vi "JPARC_foil_main.vi"() -> ()   [LabVIEW 2017]
uses:
  <vilib>/express/express arith-compare/Formula/XNode/ExpressFormulaBlockNode.xnode
  istr.lib/Agilent 33XXX Series/Agilent 33XXX Series.lvlib
panel:
  in  "Tab Control":enum32{"Main", "Debugging "}(tab)
  out "dt":dbl=0.05
  in  "Stop degauss":bool
  out "Counter":i32=600
  out "Waveform Chart":dbl(graph)
  in  "order":i64=2
  in  "Start Degauss":bool
  in  "T_end (s)":dbl=30.0 format="%_5f"
  in  "T_period (s)":dbl=1.0 format="%_5f"
  in  "I_max_d (A)":dbl=10.0 format="%_5f"
  in  "Set curet (A)":dbl min=0.0 max=120.0 format="%_5f"
  in  "OUTPUT":bool
  in  "stop":bool
  in  "I_lim_up (A)":dbl=10.1 format="%_5f"
  in  "I_lim_low (A)":dbl=-0.1 format="%_5f"
  out "Graph (Set current)":cluster{timestamp[], dbl[]}(graph)={[timestamp(3707259196.4848704 s since 1904-01-01), timestamp(3707259199.20108 s since 1904-01-01), timestamp(3707259200.17246 s since 1904-01-01), timestamp(3707259200.2159233 s since 1904-01-01), timestamp(3707259200.28732 s since 1904-01-01), timestamp(3707259200.328816 s since 1904-01-01), timestamp(3707259200.377073 s since 1904-01-01), timestamp(3707259200.420492 s since 1904-01-01), timestamp(3707259200.467496 s since 1904-01-01), timestamp(3707259200.518796 s since 1904-01-01), timestamp(3707259200.570331 s since 1904-01-01), timestamp(3707259200.620787 s since 1904-01-01), timestamp(3707259200.672 s since 1904-01-01), timestamp(3707259200.7227407 s since 1904-01-01), timestamp(3707259200.7737064 s since 1904-01-01), timestamp(3707259200.8259854 s since 1904-01-01), timestamp(3707259200.8772697 s since 1904-01-01), timestamp(3707259200.9277143 s since 1904-01-01), timestamp(3707259200.979037 s since 1904-01-01), timestamp(3707259201.0299745 s since 1904-01-01), timestamp(3707259201.081536 s since 1904-01-01), timestamp(3707259201.13187 s since 1904-01-01), timestamp(3707259201.182979 s since 1904-01-01), timestamp(3707259201.2563944 s since 1904-01-01), timestamp(3707259201.299408 s since 1904-01-01), timestamp(3707259201.342004 s since 1904-01-01), timestamp(3707259201.3879175 s since 1904-01-01), timestamp(3707259201.4399514 s since 1904-01-01), timestamp(3707259201.4893274 s since 1904-01-01), timestamp(3707259201.5397305 s since 1904-01-01), timestamp(3707259201.5915103 s since 1904-01-01), timestamp(3707259201.6417384 s since 1904-01-01), timestamp(3707259201.693012 s since 1904-01-01), timestamp(3707259201.7436895 s since 1904-01-01), timestamp(3707259201.7946744 s since 1904-01-01), timestamp(3707259201.845514 s since 1904-01-01), timestamp(3707259201.8961496 s since 1904-01-01), timestamp(3707259201.9476814 s since 1904-01-01), timestamp(3707259201.999445 s since 1904-01-01), timestamp(3707259202.0498457 s since 1904-01-01), timestamp(3707259202.101092 s since 1904-01-01), timestamp(3707259202.152056 s since 1904-01-01), timestamp(3707259202.204391 s since 1904-01-01), timestamp(3707259202.2552943 s since 1904-01-01), timestamp(3707259202.305813 s since 1904-01-01), timestamp(3707259202.3572016 s since 1904-01-01), timestamp(3707259202.408192 s since 1904-01-01), timestamp(3707259202.458596 s since 1904-01-01), timestamp(3707259202.5099535 s since 1904-01-01), timestamp(3707259202.56095 s since 1904-01-01), timestamp(3707259202.6127977 s since 1904-01-01), timestamp(3707259202.6857367 s since 1904-01-01), timestamp(3707259202.727055 s since 1904-01-01), timestamp(3707259202.77362 s since 1904-01-01), timestamp(3707259202.818931 s since 1904-01-01), timestamp(3707259202.8698378 s since 1904-01-01), timestamp(3707259202.921864 s since 1904-01-01), timestamp(3707259202.9730167 s since 1904-01-01), timestamp(3707259203.0247264 s since 1904-01-01), timestamp(3707259203.0752497 s since 1904-01-01), timestamp(3707259203.1262217 s since 1904-01-01), timestamp(3707259203.1771607 s since 1904-01-01), timestamp(3707259203.2284536 s since 1904-01-01), timestamp(3707259203.279292 s since 1904-01-01), timestamp(3707259203.3309326 s since 1904-01-01), timestamp(3707259203.3821626 s since 1904-01-01), timestamp(3707259203.4327054 s since 1904-01-01), timestamp(3707259203.4840465 s since 1904-01-01), timestamp(3707259203.5348983 s since 1904-01-01), timestamp(3707259203.586394 s since 1904-01-01), timestamp(3707259203.636896 s since 1904-01-01), timestamp(3707259203.687648 s since 1904-01-01), timestamp(3707259203.7388554 s since 1904-01-01), timestamp(3707259203.7898073 s since 1904-01-01), timestamp(3707259203.8409944 s since 1904-01-01), timestamp(3707259203.8924065 s since 1904-01-01), timestamp(3707259203.9434342 s since 1904-01-01), timestamp(3707259203.994741 s since 1904-01-01), timestamp(3707259204.046955 s since 1904-01-01), timestamp(3707259204.0980425 s since 1904-01-01), timestamp(3707259204.1488814 s since 1904-01-01), timestamp(3707259204.200164 s since 1904-01-01), timestamp(3707259204.2748857 s since 1904-01-01), timestamp(3707259204.321075 s since 1904-01-01), timestamp(3707259204.364665 s since 1904-01-01), timestamp(3707259204.410939 s since 1904-01-01), timestamp(3707259204.462568 s since 1904-01-01), timestamp(3707259204.513267 s since 1904-01-01), timestamp(3707259204.5636735 s since 1904-01-01), timestamp(3707259204.6150465 s since 1904-01-01), timestamp(3707259204.666663 s since 1904-01-01), timestamp(3707259204.7179313 s since 1904-01-01), timestamp(3707259204.7687726 s since 1904-01-01), timestamp(3707259204.819624 s since 1904-01-01), timestamp(3707259204.870779 s since 1904-01-01), timestamp(3707259204.922157 s since 1904-01-01), timestamp(3707259204.9727407 s since 1904-01-01), timestamp(3707259205.0238824 s since 1904-01-01), timestamp(3707259205.0761695 s since 1904-01-01), timestamp(3707259205.127436 s since 1904-01-01), timestamp(3707259205.177644 s since 1904-01-01), timestamp(3707259205.230016 s since 1904-01-01), timestamp(3707259205.281155 s since 1904-01-01), timestamp(3707259205.3321023 s since 1904-01-01), timestamp(3707259205.384508 s since 1904-01-01), timestamp(3707259205.4351106 s since 1904-01-01), timestamp(3707259205.4859486 s since 1904-01-01), timestamp(3707259205.537502 s since 1904-01-01), timestamp(3707259205.587603 s since 1904-01-01), timestamp(3707259205.6386504 s since 1904-01-01), timestamp(3707259205.69032 s since 1904-01-01), timestamp(3707259205.74035 s since 1904-01-01), timestamp(3707259205.791466 s since 1904-01-01), timestamp(3707259205.8418894 s since 1904-01-01), timestamp(3707259205.8925257 s since 1904-01-01), timestamp(3707259205.9429784 s since 1904-01-01), timestamp(3707259205.993564 s since 1904-01-01), timestamp(3707259206.043586 s since 1904-01-01), timestamp(3707259206.0935864 s since 1904-01-01), timestamp(3707259206.14396 s since 1904-01-01), timestamp(3707259206.194829 s since 1904-01-01), timestamp(3707259206.2456946 s since 1904-01-01), timestamp(3707259206.3135138 s since 1904-01-01), timestamp(3707259206.3546143 s since 1904-01-01), timestamp(3707259206.4024615 s since 1904-01-01), timestamp(3707259206.4513326 s since 1904-01-01), timestamp(3707259206.5024624 s since 1904-01-01), timestamp(3707259206.5528274 s since 1904-01-01), timestamp(3707259206.6034446 s since 1904-01-01), timestamp(3707259206.653367 s since 1904-01-01), timestamp(3707259206.705113 s since 1904-01-01), timestamp(3707259206.754691 s since 1904-01-01), timestamp(3707259206.806076 s since 1904-01-01), timestamp(3707259206.857049 s since 1904-01-01), timestamp(3707259206.9079337 s since 1904-01-01), timestamp(3707259206.9591393 s since 1904-01-01), timestamp(3707259207.010139 s since 1904-01-01), timestamp(3707259207.061363 s since 1904-01-01), timestamp(3707259207.1352954 s since 1904-01-01), timestamp(3707259207.1819334 s since 1904-01-01), timestamp(3707259207.227907 s since 1904-01-01), timestamp(3707259207.2730746 s since 1904-01-01), timestamp(3707259207.3175426 s since 1904-01-01), timestamp(3707259207.3691216 s since 1904-01-01), timestamp(3707259207.419863 s since 1904-01-01), timestamp(3707259207.4709153 s since 1904-01-01), timestamp(3707259207.522387 s since 1904-01-01), timestamp(3707259207.5742 s since 1904-01-01), timestamp(3707259207.626405 s since 1904-01-01), timestamp(3707259207.676672 s since 1904-01-01), timestamp(3707259207.7275534 s since 1904-01-01), timestamp(3707259207.7778554 s since 1904-01-01), timestamp(3707259207.8297663 s since 1904-01-01), timestamp(3707259207.88111 s since 1904-01-01), timestamp(3707259207.93376 s since 1904-01-01), timestamp(3707259207.9848967 s since 1904-01-01), timestamp(3707259208.0358834 s since 1904-01-01), timestamp(3707259208.087055 s since 1904-01-01), timestamp(3707259208.1377134 s since 1904-01-01), timestamp(3707259208.1888857 s since 1904-01-01), timestamp(3707259208.241416 s since 1904-01-01), timestamp(3707259208.2919464 s since 1904-01-01), timestamp(3707259208.3427296 s since 1904-01-01), timestamp(3707259208.393376 s since 1904-01-01), timestamp(3707259208.443455 s since 1904-01-01), timestamp(3707259208.4941254 s since 1904-01-01), timestamp(3707259208.5451374 s since 1904-01-01), timestamp(3707259208.596422 s since 1904-01-01), timestamp(3707259208.647224 s since 1904-01-01), timestamp(3707259208.6983647 s since 1904-01-01), timestamp(3707259208.748924 s since 1904-01-01), timestamp(3707259208.800724 s since 1904-01-01), timestamp(3707259208.851848 s since 1904-01-01), timestamp(3707259208.904263 s since 1904-01-01), timestamp(3707259208.954531 s since 1904-01-01), timestamp(3707259209.0045705 s since 1904-01-01), timestamp(3707259209.056037 s since 1904-01-01), timestamp(3707259209.107112 s since 1904-01-01), timestamp(3707259209.1579194 s since 1904-01-01), timestamp(3707259209.2093368 s since 1904-01-01), timestamp(3707259209.260172 s since 1904-01-01), timestamp(3707259209.311596 s since 1904-01-01), timestamp(3707259209.362818 s since 1904-01-01), timestamp(3707259209.4141088 s since 1904-01-01), timestamp(3707259209.4664073 s since 1904-01-01), timestamp(3707259209.517049 s since 1904-01-01), timestamp(3707259209.56796 s since 1904-01-01), timestamp(3707259209.6186466 s since 1904-01-01), timestamp(3707259209.6698775 s since 1904-01-01), timestamp(3707259209.721443 s since 1904-01-01), timestamp(3707259209.771893 s since 1904-01-01), timestamp(3707259209.8232145 s since 1904-01-01), timestamp(3707259209.87515 s since 1904-01-01), timestamp(3707259209.9262233 s since 1904-01-01), timestamp(3707259209.9767776 s since 1904-01-01), timestamp(3707259210.0292993 s since 1904-01-01), timestamp(3707259210.0800896 s since 1904-01-01), timestamp(3707259210.1313114 s since 1904-01-01), timestamp(3707259210.1819234 s since 1904-01-01), timestamp(3707259210.2327647 s since 1904-01-01), timestamp(3707259210.283632 s since 1904-01-01), timestamp(3707259210.3363066 s since 1904-01-01), timestamp(3707259210.38682 s since 1904-01-01), timestamp(3707259210.439037 s since 1904-01-01), timestamp(3707259210.489682 s since 1904-01-01), timestamp(3707259210.5407295 s since 1904-01-01), timestamp(3707259210.592229 s since 1904-01-01), timestamp(3707259210.6426926 s since 1904-01-01), timestamp(3707259210.6941586 s since 1904-01-01), timestamp(3707259210.7443247 s since 1904-01-01), timestamp(3707259210.7950273 s since 1904-01-01), timestamp(3707259210.8457465 s since 1904-01-01), timestamp(3707259210.897409 s since 1904-01-01), timestamp(3707259210.9487 s since 1904-01-01), timestamp(3707259210.9995775 s since 1904-01-01), timestamp(3707259211.050323 s since 1904-01-01), timestamp(3707259211.101493 s since 1904-01-01), timestamp(3707259211.151855 s since 1904-01-01), timestamp(3707259211.203181 s since 1904-01-01), timestamp(3707259211.2537966 s since 1904-01-01), timestamp(3707259211.3054895 s since 1904-01-01), timestamp(3707259211.355844 s since 1904-01-01), timestamp(3707259211.4072433 s since 1904-01-01), timestamp(3707259211.4580126 s since 1904-01-01), timestamp(3707259211.5096097 s since 1904-01-01), timestamp(3707259211.560656 s since 1904-01-01), timestamp(3707259211.611928 s since 1904-01-01), timestamp(3707259211.6628976 s since 1904-01-01), timestamp(3707259211.714095 s since 1904-01-01), timestamp(3707259211.766273 s since 1904-01-01), timestamp(3707259211.8179936 s since 1904-01-01), timestamp(3707259211.869491 s since 1904-01-01), timestamp(3707259211.921025 s since 1904-01-01), timestamp(3707259211.972306 s since 1904-01-01), timestamp(3707259212.023468 s since 1904-01-01), timestamp(3707259212.0753655 s since 1904-01-01), timestamp(3707259212.126084 s since 1904-01-01), timestamp(3707259212.1770864 s since 1904-01-01), timestamp(3707259212.229044 s since 1904-01-01), timestamp(3707259212.2800536 s since 1904-01-01), timestamp(3707259212.3323584 s since 1904-01-01), timestamp(3707259212.383467 s since 1904-01-01), timestamp(3707259212.4347086 s since 1904-01-01), timestamp(3707259212.486989 s since 1904-01-01), timestamp(3707259212.53818 s since 1904-01-01), timestamp(3707259212.58933 s since 1904-01-01), timestamp(3707259212.640089 s since 1904-01-01), timestamp(3707259212.701696 s since 1904-01-01), timestamp(3707259212.7540417 s since 1904-01-01), timestamp(3707259212.8061337 s since 1904-01-01), timestamp(3707259212.8567905 s since 1904-01-01), timestamp(3707259212.9081287 s since 1904-01-01), timestamp(3707259212.9602423 s since 1904-01-01), timestamp(3707259213.0107985 s since 1904-01-01), timestamp(3707259213.063319 s since 1904-01-01), timestamp(3707259213.1145 s since 1904-01-01), timestamp(3707259213.165478 s since 1904-01-01), timestamp(3707259213.216491 s since 1904-01-01), timestamp(3707259213.267567 s since 1904-01-01), timestamp(3707259213.318584 s since 1904-01-01), timestamp(3707259213.3694696 s since 1904-01-01), timestamp(3707259213.4201455 s since 1904-01-01), timestamp(3707259213.4707623 s since 1904-01-01), timestamp(3707259213.5227647 s since 1904-01-01), timestamp(3707259213.5735393 s since 1904-01-01), timestamp(3707259213.6239495 s since 1904-01-01), timestamp(3707259213.675685 s since 1904-01-01), timestamp(3707259213.7274256 s since 1904-01-01), timestamp(3707259213.7781906 s since 1904-01-01), timestamp(3707259213.8294616 s since 1904-01-01), timestamp(3707259213.880292 s since 1904-01-01), timestamp(3707259213.9308977 s since 1904-01-01), timestamp(3707259213.982133 s since 1904-01-01), timestamp(3707259214.0334015 s since 1904-01-01), timestamp(3707259214.084085 s since 1904-01-01), timestamp(3707259214.135271 s since 1904-01-01), timestamp(3707259214.185329 s since 1904-01-01), timestamp(3707259214.2361574 s since 1904-01-01), timestamp(3707259214.287383 s since 1904-01-01), timestamp(3707259214.337472 s since 1904-01-01), timestamp(3707259214.3874817 s since 1904-01-01), timestamp(3707259214.438272 s since 1904-01-01), timestamp(3707259214.489022 s since 1904-01-01), timestamp(3707259214.540349 s since 1904-01-01), timestamp(3707259214.590536 s since 1904-01-01), timestamp(3707259214.64076 s since 1904-01-01), timestamp(3707259214.700007 s since 1904-01-01), timestamp(3707259214.7501864 s since 1904-01-01), timestamp(3707259214.8015146 s since 1904-01-01), timestamp(3707259214.8524246 s since 1904-01-01), timestamp(3707259214.9026446 s since 1904-01-01), timestamp(3707259214.954119 s since 1904-01-01), timestamp(3707259215.0048494 s since 1904-01-01), timestamp(3707259215.057986 s since 1904-01-01), timestamp(3707259215.10916 s since 1904-01-01), timestamp(3707259215.1601553 s since 1904-01-01), timestamp(3707259215.213757 s since 1904-01-01), timestamp(3707259215.265211 s since 1904-01-01), timestamp(3707259215.316068 s since 1904-01-01), timestamp(3707259215.3673697 s since 1904-01-01), timestamp(3707259215.417912 s since 1904-01-01), timestamp(3707259215.469684 s since 1904-01-01), timestamp(3707259215.520413 s since 1904-01-01), timestamp(3707259215.570737 s since 1904-01-01), timestamp(3707259215.621899 s since 1904-01-01), timestamp(3707259215.672473 s since 1904-01-01), timestamp(3707259215.7224584 s since 1904-01-01), timestamp(3707259215.773552 s since 1904-01-01), timestamp(3707259215.824029 s since 1904-01-01), timestamp(3707259215.8763375 s since 1904-01-01), timestamp(3707259215.927059 s since 1904-01-01), timestamp(3707259215.9783382 s since 1904-01-01), timestamp(3707259216.0288734 s since 1904-01-01), timestamp(3707259216.0800967 s since 1904-01-01), timestamp(3707259216.1305 s since 1904-01-01), timestamp(3707259216.1806087 s since 1904-01-01), timestamp(3707259216.2318783 s since 1904-01-01), timestamp(3707259216.283163 s since 1904-01-01), timestamp(3707259216.3337545 s since 1904-01-01), timestamp(3707259216.3863034 s since 1904-01-01), timestamp(3707259216.436903 s since 1904-01-01), timestamp(3707259216.4876494 s since 1904-01-01), timestamp(3707259216.5379634 s since 1904-01-01), timestamp(3707259216.5895176 s since 1904-01-01), timestamp(3707259216.640459 s since 1904-01-01), timestamp(3707259216.690654 s since 1904-01-01), timestamp(3707259216.742255 s since 1904-01-01), timestamp(3707259216.7949896 s since 1904-01-01), timestamp(3707259216.8460145 s since 1904-01-01), timestamp(3707259216.8970914 s since 1904-01-01), timestamp(3707259216.9476047 s since 1904-01-01), timestamp(3707259217.0005393 s since 1904-01-01), timestamp(3707259217.051352 s since 1904-01-01), timestamp(3707259217.102024 s since 1904-01-01), timestamp(3707259217.1528993 s since 1904-01-01), timestamp(3707259217.203648 s since 1904-01-01), timestamp(3707259217.256073 s since 1904-01-01), timestamp(3707259217.3070145 s since 1904-01-01), timestamp(3707259217.356732 s since 1904-01-01), timestamp(3707259217.4104424 s since 1904-01-01), timestamp(3707259217.4607873 s since 1904-01-01), timestamp(3707259217.5116177 s since 1904-01-01), timestamp(3707259217.5639296 s since 1904-01-01), timestamp(3707259217.6161304 s since 1904-01-01), timestamp(3707259217.6665506 s since 1904-01-01), timestamp(3707259217.7166615 s since 1904-01-01), timestamp(3707259217.767932 s since 1904-01-01), timestamp(3707259217.819317 s since 1904-01-01), timestamp(3707259217.8699727 s since 1904-01-01), timestamp(3707259217.9206257 s since 1904-01-01), timestamp(3707259217.9714575 s since 1904-01-01), timestamp(3707259218.021664 s since 1904-01-01), timestamp(3707259218.0726857 s since 1904-01-01), timestamp(3707259218.124248 s since 1904-01-01), timestamp(3707259218.1760406 s since 1904-01-01), timestamp(3707259218.2275505 s since 1904-01-01), timestamp(3707259218.2780695 s since 1904-01-01), timestamp(3707259218.3291097 s since 1904-01-01), timestamp(3707259218.3796663 s since 1904-01-01), timestamp(3707259218.4309096 s since 1904-01-01), timestamp(3707259218.482177 s since 1904-01-01), timestamp(3707259218.5334377 s since 1904-01-01), timestamp(3707259218.5839825 s since 1904-01-01), timestamp(3707259218.6347857 s since 1904-01-01), timestamp(3707259218.687488 s since 1904-01-01), timestamp(3707259218.7368326 s since 1904-01-01), timestamp(3707259218.7891154 s since 1904-01-01), timestamp(3707259218.840208 s since 1904-01-01), timestamp(3707259218.891742 s since 1904-01-01), timestamp(3707259218.94312 s since 1904-01-01), timestamp(3707259218.9935336 s since 1904-01-01), timestamp(3707259219.0437903 s since 1904-01-01), timestamp(3707259219.095799 s since 1904-01-01), timestamp(3707259219.155056 s since 1904-01-01), timestamp(3707259219.2061977 s since 1904-01-01), timestamp(3707259219.266284 s since 1904-01-01), timestamp(3707259219.317372 s since 1904-01-01), timestamp(3707259219.367924 s since 1904-01-01), timestamp(3707259219.4185576 s since 1904-01-01), timestamp(3707259219.4702945 s since 1904-01-01), timestamp(3707259219.520776 s since 1904-01-01), timestamp(3707259219.5729456 s since 1904-01-01), timestamp(3707259219.6249 s since 1904-01-01), timestamp(3707259219.676088 s since 1904-01-01), timestamp(3707259219.726608 s since 1904-01-01), timestamp(3707259219.7775393 s since 1904-01-01), timestamp(3707259219.8276463 s since 1904-01-01), timestamp(3707259219.8794065 s since 1904-01-01), timestamp(3707259219.9297304 s since 1904-01-01), timestamp(3707259219.981024 s since 1904-01-01), timestamp(3707259220.032031 s since 1904-01-01), timestamp(3707259220.08276 s since 1904-01-01), timestamp(3707259220.13502 s since 1904-01-01), timestamp(3707259220.186343 s since 1904-01-01), timestamp(3707259220.2370896 s since 1904-01-01), timestamp(3707259220.2879705 s since 1904-01-01), timestamp(3707259220.340339 s since 1904-01-01), timestamp(3707259220.391716 s since 1904-01-01), timestamp(3707259220.450717 s since 1904-01-01), timestamp(3707259220.503291 s since 1904-01-01), timestamp(3707259220.5555534 s since 1904-01-01), timestamp(3707259220.606714 s since 1904-01-01), timestamp(3707259220.658076 s since 1904-01-01), timestamp(3707259220.709576 s since 1904-01-01), timestamp(3707259220.759384 s since 1904-01-01), timestamp(3707259220.810531 s since 1904-01-01), timestamp(3707259220.860863 s since 1904-01-01), timestamp(3707259220.9124303 s since 1904-01-01), timestamp(3707259220.9629617 s since 1904-01-01), timestamp(3707259221.01416 s since 1904-01-01), timestamp(3707259221.0653095 s since 1904-01-01), timestamp(3707259221.115598 s since 1904-01-01), timestamp(3707259221.1672006 s since 1904-01-01), timestamp(3707259221.217863 s since 1904-01-01), timestamp(3707259221.2699904 s since 1904-01-01), timestamp(3707259221.322552 s since 1904-01-01), timestamp(3707259221.3738728 s since 1904-01-01), timestamp(3707259221.425934 s since 1904-01-01), timestamp(3707259221.477443 s since 1904-01-01), timestamp(3707259221.52782 s since 1904-01-01), timestamp(3707259221.5785017 s since 1904-01-01), timestamp(3707259221.628906 s since 1904-01-01), timestamp(3707259221.6805334 s since 1904-01-01), timestamp(3707259221.7307234 s since 1904-01-01), timestamp(3707259221.7821255 s since 1904-01-01), timestamp(3707259221.833152 s since 1904-01-01), timestamp(3707259221.883951 s since 1904-01-01), timestamp(3707259221.9346166 s since 1904-01-01), timestamp(3707259221.987086 s since 1904-01-01), timestamp(3707259222.0374384 s since 1904-01-01), timestamp(3707259222.087833 s since 1904-01-01), timestamp(3707259222.1391544 s since 1904-01-01), timestamp(3707259222.1914062 s since 1904-01-01), timestamp(3707259222.2418942 s since 1904-01-01), timestamp(3707259222.2929454 s since 1904-01-01), timestamp(3707259222.3446894 s since 1904-01-01), timestamp(3707259222.3967385 s since 1904-01-01), timestamp(3707259222.447489 s since 1904-01-01), timestamp(3707259222.497763 s since 1904-01-01), timestamp(3707259222.54918 s since 1904-01-01), timestamp(3707259222.6010094 s since 1904-01-01), timestamp(3707259222.6523314 s since 1904-01-01), timestamp(3707259222.7027655 s since 1904-01-01), timestamp(3707259222.754297 s since 1904-01-01), timestamp(3707259222.8053575 s since 1904-01-01), timestamp(3707259222.856412 s since 1904-01-01), timestamp(3707259222.9070864 s since 1904-01-01), timestamp(3707259222.958297 s since 1904-01-01), timestamp(3707259223.009618 s since 1904-01-01), timestamp(3707259223.0613146 s since 1904-01-01), timestamp(3707259223.11218 s since 1904-01-01), timestamp(3707259223.1625433 s since 1904-01-01), timestamp(3707259223.2127657 s since 1904-01-01), timestamp(3707259223.2645383 s since 1904-01-01), timestamp(3707259223.3150783 s since 1904-01-01), timestamp(3707259223.3659673 s since 1904-01-01), timestamp(3707259223.418496 s since 1904-01-01), timestamp(3707259223.4693246 s since 1904-01-01), timestamp(3707259223.5205846 s since 1904-01-01), timestamp(3707259223.570944 s since 1904-01-01), timestamp(3707259223.6216254 s since 1904-01-01), timestamp(3707259223.682088 s since 1904-01-01), timestamp(3707259223.733576 s since 1904-01-01), timestamp(3707259223.784137 s since 1904-01-01), timestamp(3707259223.83652 s since 1904-01-01), timestamp(3707259223.8887234 s since 1904-01-01), timestamp(3707259223.939524 s since 1904-01-01), timestamp(3707259223.990504 s since 1904-01-01), timestamp(3707259224.0408306 s since 1904-01-01), timestamp(3707259224.093295 s since 1904-01-01), timestamp(3707259224.1437054 s since 1904-01-01), timestamp(3707259224.19502 s since 1904-01-01), timestamp(3707259224.245454 s since 1904-01-01), timestamp(3707259224.29636 s since 1904-01-01), timestamp(3707259224.347352 s since 1904-01-01), timestamp(3707259224.398108 s since 1904-01-01), timestamp(3707259224.449426 s since 1904-01-01), timestamp(3707259224.500648 s since 1904-01-01), timestamp(3707259224.5518937 s since 1904-01-01), timestamp(3707259224.6029873 s since 1904-01-01), timestamp(3707259224.654089 s since 1904-01-01), timestamp(3707259224.706424 s since 1904-01-01), timestamp(3707259224.75725 s since 1904-01-01), timestamp(3707259224.8075743 s since 1904-01-01), timestamp(3707259224.857317 s since 1904-01-01), timestamp(3707259224.908 s since 1904-01-01), timestamp(3707259224.9592695 s since 1904-01-01), timestamp(3707259225.0099897 s since 1904-01-01), timestamp(3707259225.060612 s since 1904-01-01), timestamp(3707259225.1121006 s since 1904-01-01), timestamp(3707259225.163561 s since 1904-01-01), timestamp(3707259225.2141614 s since 1904-01-01), timestamp(3707259225.2663345 s since 1904-01-01), timestamp(3707259225.316788 s since 1904-01-01), timestamp(3707259225.3684354 s since 1904-01-01), timestamp(3707259225.419561 s since 1904-01-01), timestamp(3707259225.4698944 s since 1904-01-01), timestamp(3707259225.52236 s since 1904-01-01), timestamp(3707259225.5731654 s since 1904-01-01), timestamp(3707259225.624091 s since 1904-01-01), timestamp(3707259225.675978 s since 1904-01-01), timestamp(3707259225.727556 s since 1904-01-01), timestamp(3707259225.778472 s since 1904-01-01), timestamp(3707259225.8297086 s since 1904-01-01), timestamp(3707259225.8806744 s since 1904-01-01), timestamp(3707259225.9340096 s since 1904-01-01), timestamp(3707259225.9844646 s since 1904-01-01), timestamp(3707259226.0369096 s since 1904-01-01), timestamp(3707259226.088491 s since 1904-01-01), timestamp(3707259226.138916 s since 1904-01-01), timestamp(3707259226.1902647 s since 1904-01-01), timestamp(3707259226.241206 s since 1904-01-01), timestamp(3707259226.29248 s since 1904-01-01), timestamp(3707259226.3426905 s since 1904-01-01), timestamp(3707259226.393713 s since 1904-01-01), timestamp(3707259226.4446816 s since 1904-01-01), timestamp(3707259226.4961057 s since 1904-01-01), timestamp(3707259226.5475063 s since 1904-01-01), timestamp(3707259226.5974383 s since 1904-01-01), timestamp(3707259226.647401 s since 1904-01-01), timestamp(3707259226.6976 s since 1904-01-01), timestamp(3707259226.748803 s since 1904-01-01), timestamp(3707259226.8003407 s since 1904-01-01), timestamp(3707259226.8516073 s since 1904-01-01), timestamp(3707259226.9029126 s since 1904-01-01), timestamp(3707259226.95415 s since 1904-01-01), timestamp(3707259227.0043664 s since 1904-01-01), timestamp(3707259227.055092 s since 1904-01-01), timestamp(3707259227.1056786 s since 1904-01-01), timestamp(3707259227.15715 s since 1904-01-01), timestamp(3707259227.2084703 s since 1904-01-01), timestamp(3707259227.2600713 s since 1904-01-01), timestamp(3707259227.3114734 s since 1904-01-01), timestamp(3707259227.36184 s since 1904-01-01), timestamp(3707259227.41304 s since 1904-01-01), timestamp(3707259227.4637184 s since 1904-01-01), timestamp(3707259227.516283 s since 1904-01-01), timestamp(3707259227.5666585 s since 1904-01-01), timestamp(3707259227.617522 s since 1904-01-01), timestamp(3707259227.667171 s since 1904-01-01), timestamp(3707259227.717443 s since 1904-01-01), timestamp(3707259227.7677736 s since 1904-01-01), timestamp(3707259227.8190265 s since 1904-01-01), timestamp(3707259227.86989 s since 1904-01-01), timestamp(3707259227.9213367 s since 1904-01-01), timestamp(3707259227.972058 s since 1904-01-01), timestamp(3707259228.022944 s since 1904-01-01), timestamp(3707259228.0737743 s since 1904-01-01), timestamp(3707259228.126157 s since 1904-01-01), timestamp(3707259228.179792 s since 1904-01-01), timestamp(3707259228.230928 s since 1904-01-01), timestamp(3707259228.2822247 s since 1904-01-01), timestamp(3707259228.3334584 s since 1904-01-01), timestamp(3707259228.3851233 s since 1904-01-01), timestamp(3707259228.4358015 s since 1904-01-01), timestamp(3707259228.487086 s since 1904-01-01), timestamp(3707259228.5382576 s since 1904-01-01), timestamp(3707259228.589992 s since 1904-01-01), timestamp(3707259228.6409473 s since 1904-01-01), timestamp(3707259228.6921864 s since 1904-01-01), timestamp(3707259228.7431855 s since 1904-01-01), timestamp(3707259228.793529 s since 1904-01-01), timestamp(3707259228.8443007 s since 1904-01-01), timestamp(3707259228.895092 s since 1904-01-01), timestamp(3707259228.9469104 s since 1904-01-01), timestamp(3707259228.9980783 s since 1904-01-01), timestamp(3707259229.0492735 s since 1904-01-01), timestamp(3707259229.0995064 s since 1904-01-01), timestamp(3707259229.150301 s since 1904-01-01), timestamp(3707259229.201368 s since 1904-01-01), timestamp(3707259229.254064 s since 1904-01-01), timestamp(3707259229.3044486 s since 1904-01-01), timestamp(3707259229.3551073 s since 1904-01-01), timestamp(3707259229.4070864 s since 1904-01-01), timestamp(3707259229.457599 s since 1904-01-01), timestamp(3707259229.5088544 s since 1904-01-01), timestamp(3707259229.5599866 s since 1904-01-01), timestamp(3707259229.6109066 s since 1904-01-01), timestamp(3707259229.662153 s since 1904-01-01), timestamp(3707259229.712928 s since 1904-01-01), timestamp(3707259229.764052 s since 1904-01-01), timestamp(3707259229.815863 s since 1904-01-01), timestamp(3707259229.867405 s since 1904-01-01), timestamp(3707259229.916816 s since 1904-01-01), timestamp(3707259229.967896 s since 1904-01-01), timestamp(3707259230.020653 s since 1904-01-01), timestamp(3707259230.0722766 s since 1904-01-01), timestamp(3707259230.1225095 s since 1904-01-01), timestamp(3707259230.1731434 s since 1904-01-01), timestamp(3707259230.224079 s since 1904-01-01), timestamp(3707259230.2750993 s since 1904-01-01), timestamp(3707259230.3256216 s since 1904-01-01), timestamp(3707259230.3771567 s since 1904-01-01), timestamp(3707259230.427674 s since 1904-01-01), timestamp(3707259230.4784455 s since 1904-01-01), timestamp(3707259230.529454 s since 1904-01-01), timestamp(3707259230.5793514 s since 1904-01-01), timestamp(3707259230.629626 s since 1904-01-01), timestamp(3707259230.680669 s since 1904-01-01), timestamp(3707259230.7320294 s since 1904-01-01), timestamp(3707259230.7828393 s since 1904-01-01), timestamp(3707259230.834331 s since 1904-01-01), timestamp(3707259230.886357 s since 1904-01-01), timestamp(3707259230.936435 s since 1904-01-01)], array[604 elements]} caption="XY Graph"
  in  "VISA (Agilent 34402)":refnum<visa-resource-name>="GPIB0::15::INSTR"
  out "Agilent\nIntialized?":bool=TRUE
  in  "Initialize (Agilent)":bool
  in  "base path":path=path "C:/LabVIEW/DATA/J-PARC_202107/test_0623"
  out "time elapsed (ms)":u32=30726
  out "File Error Out":errorcluster
  out "error out (Agilent)":errorcluster
  # "GP016-10 control"
  # "Degaussing routine"
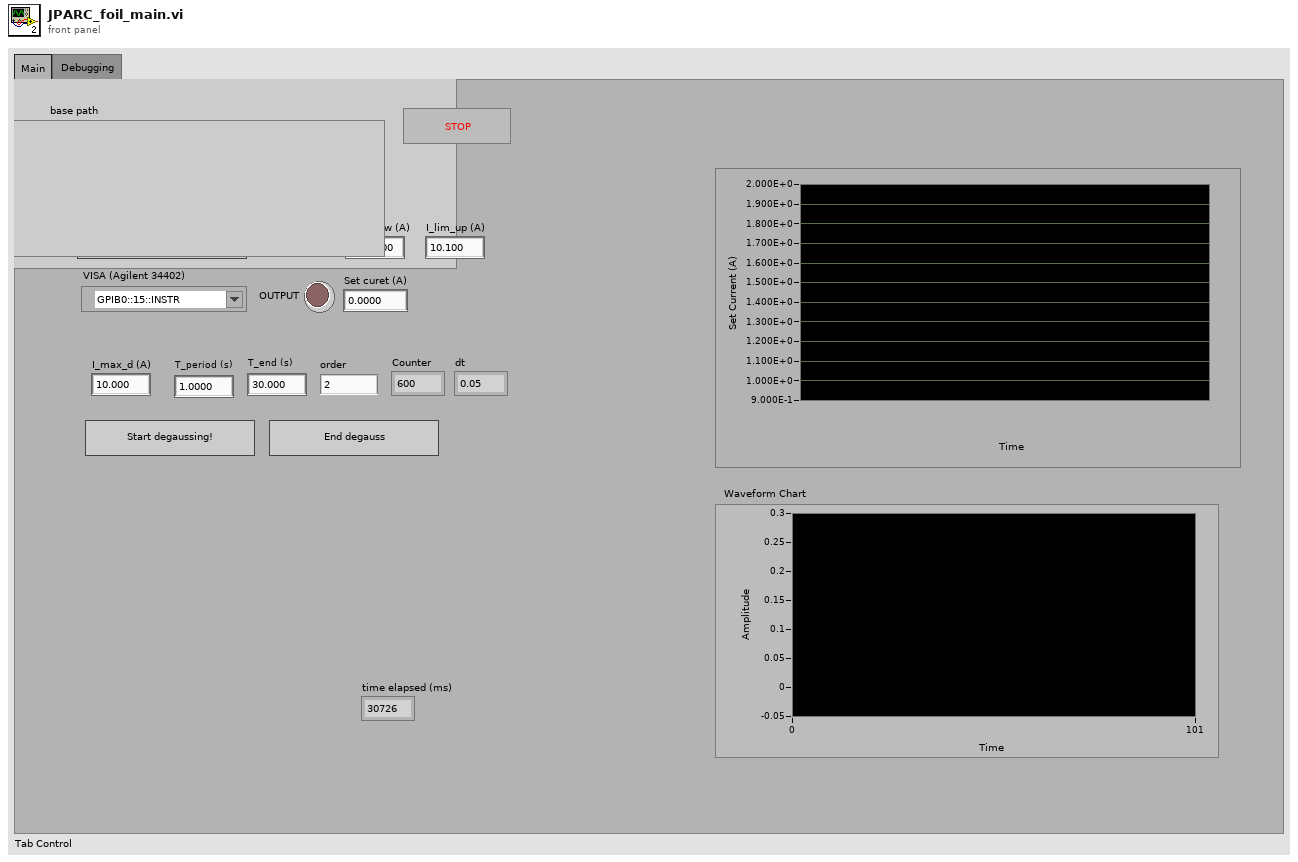
[diagram p1: front panel]
types:
  T1 = enum16{"open", "replace", "create", "open or create", "replace or create", "replace or create with confirmation"}
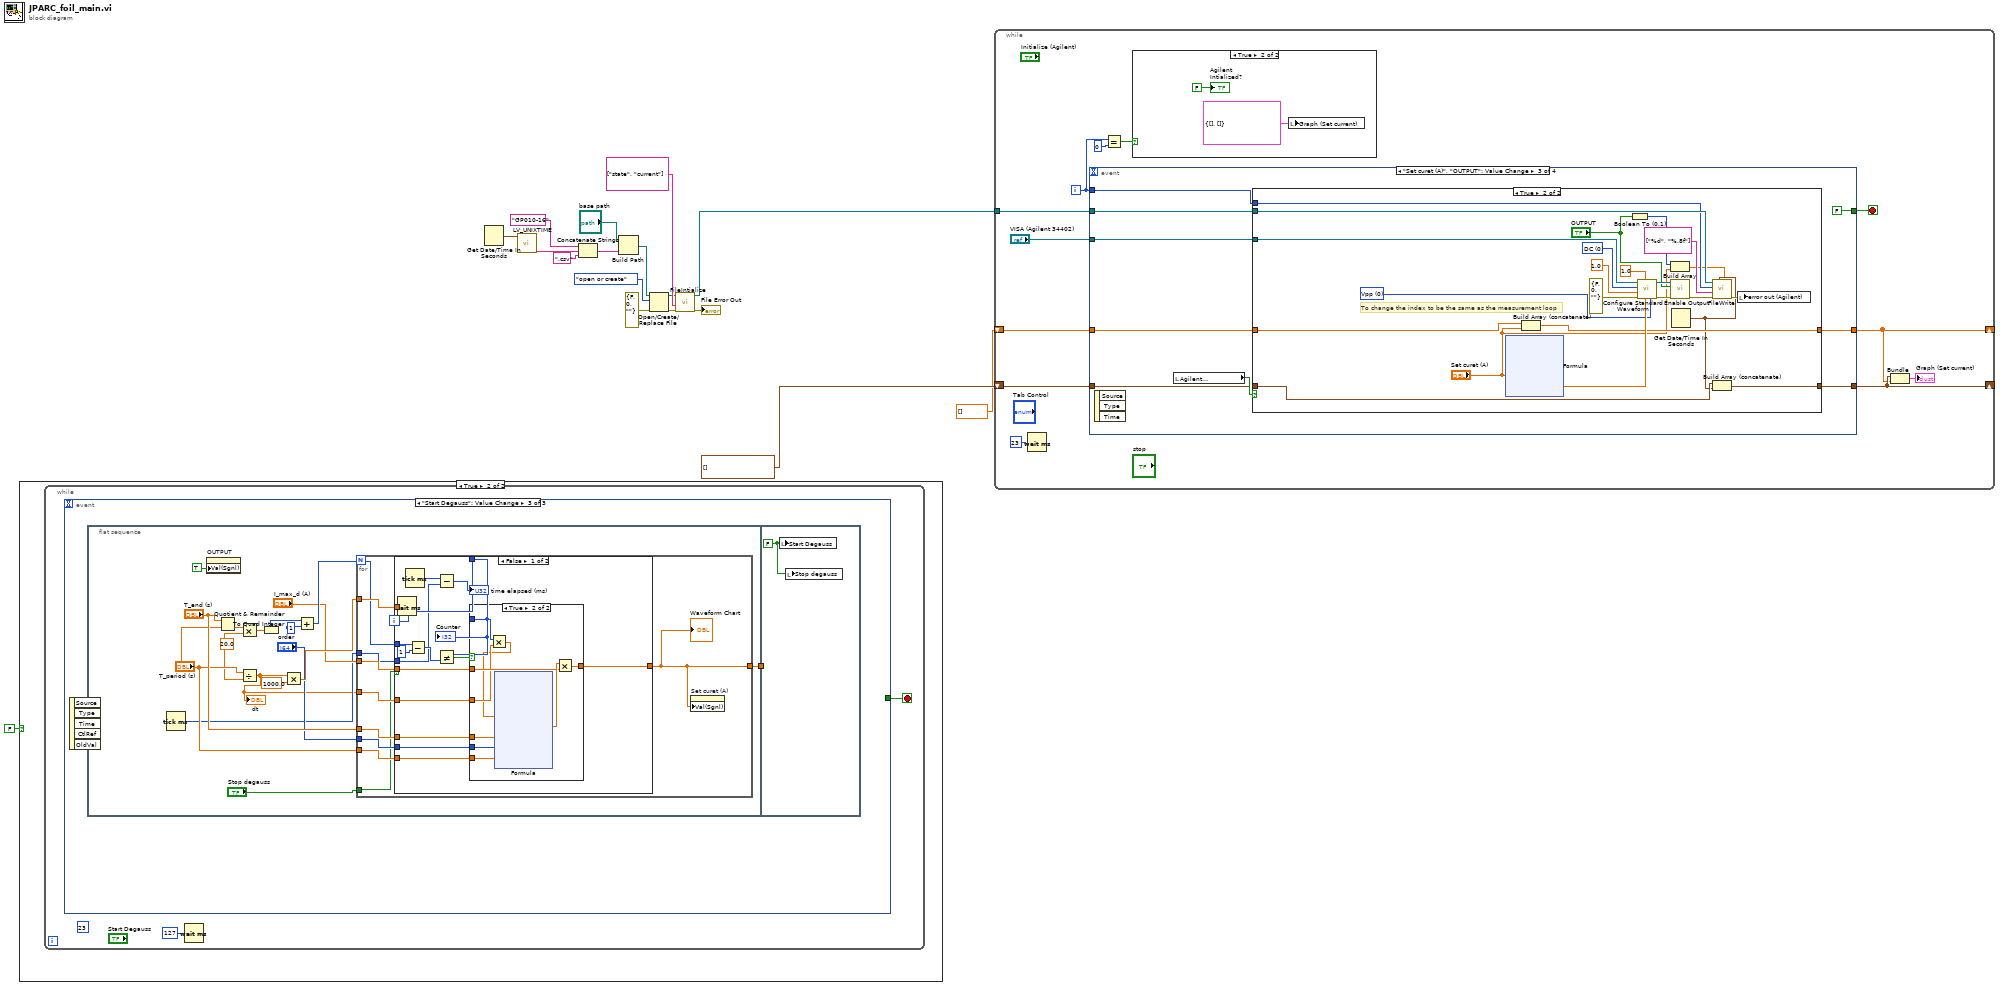
[diagram p0: block diagram]
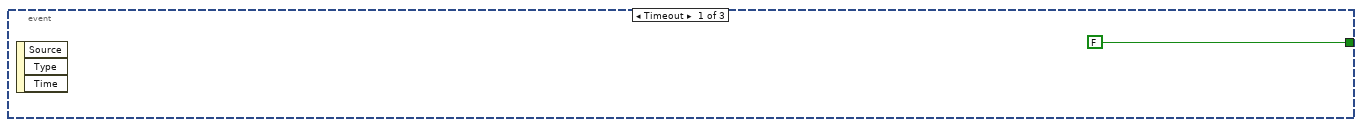
[diagram p3: hidden frame]
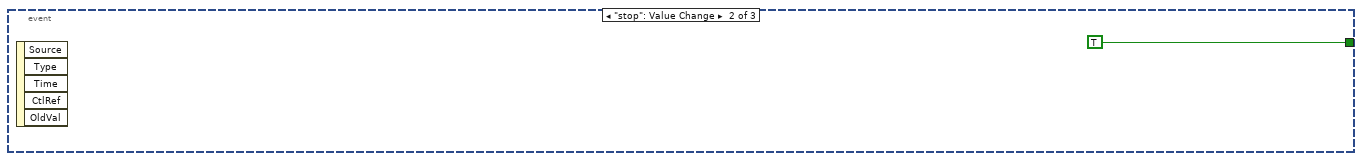
[diagram p4: hidden frame]
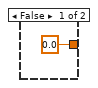
[diagram p5: hidden frame]
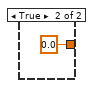
[diagram p6: hidden frame]
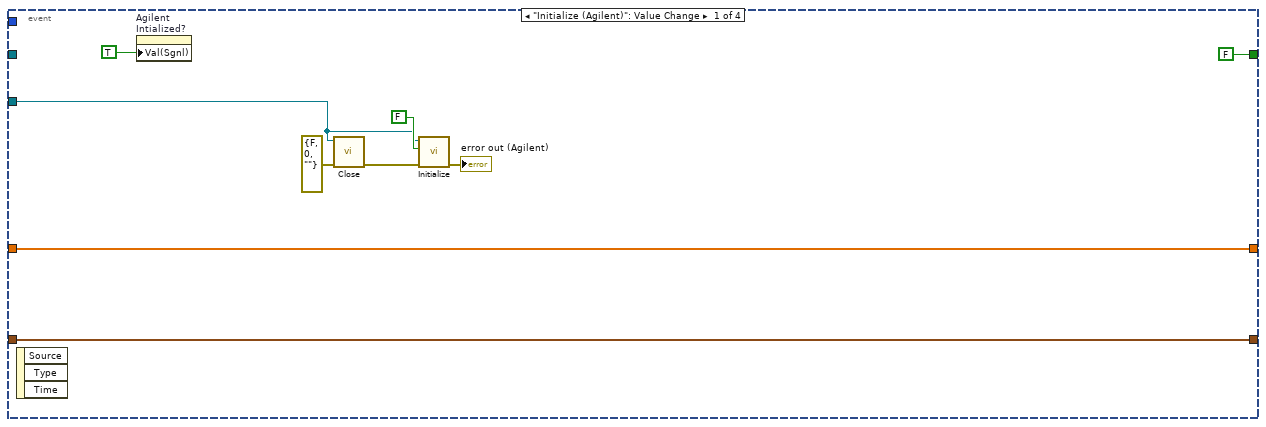
[diagram p8: hidden frame]
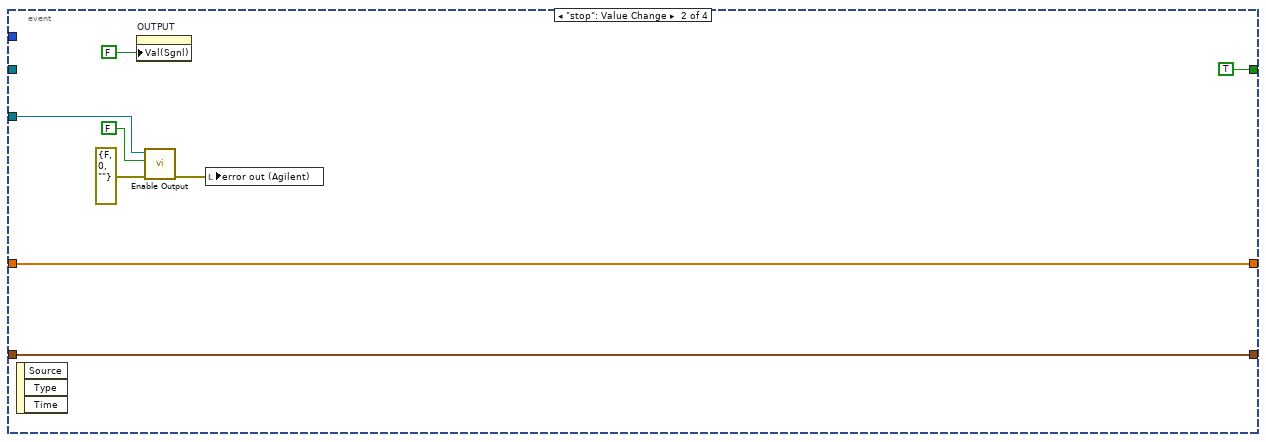
[diagram p9: hidden frame]
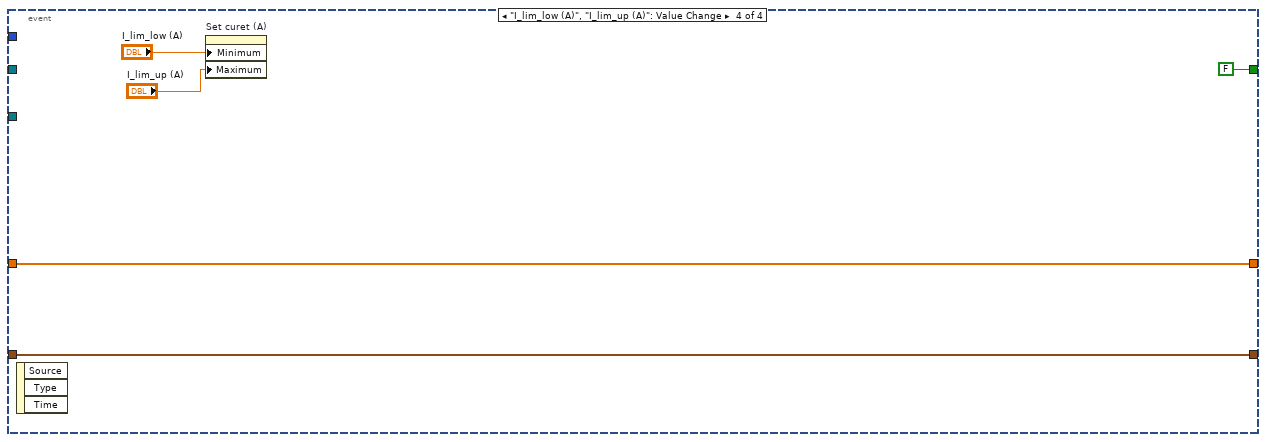
[diagram p11: hidden frame]
diagram:
  n1 = case shown="True" FALSE {
    frame False {
    }
    frame True {
      n2 = while {
        stop <- w18 stop-if-true
        (unwired) u32 23 ("milliseconds to wait")
        n3 = event shown="[2] \"Start Degauss\": Value Change" {
          selector: _ -> [_ _ _]
          dyn-events: _ -> [_ _ _]
          timeout: _ -> [_ _ _]
          tunnel: [FALSE TRUE _] -> w18
          event Timeout {
            n4 = event-data() -> ()  [unwired: 1 in, 3 out]
          }
          event "stop": Value Change {
            n5 = event-data() -> ()  [unwired: 1 in, 5 out]
          }
          event "Start Degauss": Value Change {
            n6 = event-data() -> ()  [unwired: 1 in, 5 out]
            n7 = flat-sequence {
              tunnel: [w24] -> w22
              tunnel: w22 -> [_]
              frame #0 {
                w28 = 20.0 ("y")
                n8 = Tick Count (ms)() -> (millisecond timer value=w27:u32)
                n9 = property on="OUTPUT" class="Bool (strict)"("Val(Sgnl)"=TRUE ("Value (Signaling)")) -> ()  [unwired: 2 in, 2 out]
                n10 = Quotient & Remainder(x="T_end (s)", y="T_period (s)") -> (floor(x/y)=w30:dbl)  [unwired: 1 out]
                n11 = Multiply(x=w30, y=w28) -> (x*y=w29:dbl)
                n12 = Divide(x="T_period (s)", y=w28) -> (x/y=w26:dbl)
                "dt" <- w26
                n13 = To Quad Integer(1:w29) -> (0:w38:i64)
                n14 = Multiply(x=w26, y=1000.0) -> (x*y=w35:dbl)
                n15 = Add(x=w38, y=i64 1) -> (x+y=w36:i64)
                n16 = for {
                  N: w36 -> [w44]
                  tunnel: w35 -> [w50]
                  tunnel: "T_end (s)" -> [w49]
                  tunnel: "T_period (s)" -> [w48]
                  tunnel: "order" -> [w47]
                  tunnel: "I_max_d (A)" -> [w46]
                  tunnel: w27 -> [w43]
                  tunnel: w26 -> [w42]
                  tunnel: "Stop degauss" -> [w41]
                  tunnel: [w40] -> w24
                  i -> [w45]
                  n17 = case shown="False" w41 {
                    tunnel: w50 -> [w65 _]
                    tunnel: w49 -> [w64 _]
                    tunnel: w48 -> [w63 _]
                    tunnel: w47 -> [w62 _]
                    tunnel: w46 -> [w61 _]
                    tunnel: w45 -> [w60 _]
                    tunnel: w44 -> [w58 _]
                    tunnel: w43 -> [w54 _]
                    tunnel: w42 -> [w52 _]
                    tunnel: [w51 0.0] -> w40
                    frame False {
                      n18 = Wait (ms)(milliseconds to wait=w65) -> ()  [unwired: 1 out]
                      n19 = Tick Count (ms)() -> (millisecond timer value=w55:u32)
                      n20 = Subtract(x=w58, y=1) -> (x-y=w57:i32)
                      n21 = Subtract(x=w55, y=w54) -> (x-y=→"time elapsed (ms)":u32)
                      n22 = Not Equal?(x=w60, y=w57) -> (x != y?=w59:bool)
                      n23 = case shown="True" w59 {
                        tunnel: w64 -> [_ w75]
                        tunnel: w63 -> [_ w74]
                        tunnel: w62 -> [_ w73]
                        tunnel: w60 -> [_ w69]
                        tunnel: w61 -> [_ w71]
                        tunnel: [0.0 w70] -> w51
                        tunnel: w52 -> [_ w68]
                        frame False {
                        }
                        frame True {
                          n24 = Multiply(x=w69, y=w68) -> (x*y=w67:dbl)
                          n25 = xnode "Formula"("t"=w67, "T"=w75, "m"=w73, "Tp"=w74) -> ("Result"=w72:dbl)  [unwired: 1 in, 1 out]
                          n26 = Multiply(x=w72, y=w71) -> (x*y=w70:dbl)
                        }
                      }
                      "Counter" <- w60
                    }
                    frame True {
                    }
                  }
                  "Waveform Chart" <- w40
                  n27 = property on="Set curet (A)" class="DigNum (strict)"("Val(Sgnl)"=w40) -> ()  [unwired: 2 in, 2 out]
                }
              }
              frame #1 {
                w91 = FALSE ("Start Degauss")
                n28 = local write "Start Degauss"(w91) -> ()
                n29 = local write "Stop degauss"(w91) -> ()
              }
            }
          }
        }
        n30 = Wait (ms)(milliseconds to wait=u32 127) -> ()  [unwired: 1 out]
      }
    }
  }
  n31 = Get Date/Time In Seconds() -> (seconds since 1Jan1904=w14:timestamp)
  n32 = call "LV_UNIXTIME.vi"("current time"=w14) -> ("date/time string"=w11:string)  [unwired: 9 in, 1 out]
  n33 = Concatenate Strings("GP010-16" ("name or relative path"), w11, ".csv" ("string")) -> (w9:string)
  n34 = Build Path(base path="base path", name or relative path=w9) -> (appended path=w13:path)
  n35 = Open/Create/Replace File(file path (use dialog)=w13, error in=errorcluster {"status"=FALSE, "code"=0, "source"=""}, operation (0:open)=T1."open or create") -> (refnum out=w5:refnum<file>, error out=w6:errorcluster)  [unwired: 3 in, 1 out]
  n36 = call "FileIntialize.vi"("Error In"=w6, "Labels"=string[] ["state", "current"], "refnum in"=w5) -> ("Error Out"=→"File Error Out":errorcluster, "File Refnum"=w2:refnum<file>)  [unwired: 7 in]
  n37 = while {
    shift-right: [w98] -> _
    shift-left: timestamp[] [] -> [w100]
    shift-right: [w97] -> _
    shift-left: dbl[] [] -> [w99]
    tunnel: w2 -> [w93]
    i -> [w92]
    stop <- w102 stop-if-true
    n38 = Wait (ms)(milliseconds to wait=u32 23) -> ()  [unwired: 1 out]
    n39 = event shown="[2] \"Set curet (A)\", \"OUTPUT\": Value Change" {
      selector: _ -> [_ _ _ _]
      dyn-events: _ -> [_ _ _ _]
      timeout: _ -> [_ _ _ _]
      tunnel: [FALSE ("Value (Signaling)") TRUE ("Value (Signaling)") FALSE ("Value (Signaling)") FALSE ("Value (Signaling)")] -> w102
      tunnel: "VISA (Agilent 34402)" -> [w107 w120 w129 _]
      tunnel: [w110 w115 w128 w165] -> w98
      tunnel: w100 -> [w110 w115 w127 w165]
      tunnel: [w111 w116 w126 w166] -> w97
      tunnel: w99 -> [w111 w116 w125 w166]
      tunnel: w93 -> [_ _ w124 _]
      tunnel: w92 -> [_ _ w123 _]
      event "Initialize (Agilent)": Value Change {
        n40 = event-data() -> ()  [unwired: 1 in, 3 out]
        n41 = property on="Agilent\nIntialized?" class="Bool (strict)"("Val(Sgnl)"=TRUE ("Value (Signaling)")) -> ()  [unwired: 2 in, 2 out]
        n42 = call "Close.vi"("error in (no error)"=errorcluster {"status"=FALSE, "code"=0, "source"=""}, "VISA resource name"=w107) -> ("error out"=w106:errorcluster)  [unwired: 9 in]
        n43 = call "Initialize.vi"("error in (no error)"=w106, "ID Query (True)"=FALSE, "VISA resource name"=w107) -> ("error out"=→"error out (Agilent)":errorcluster)  [unwired: 7 in, 1 out]
      }
      event "stop": Value Change {
        n44 = event-data() -> ()  [unwired: 1 in, 3 out]
        n45 = property on="OUTPUT" class="Bool (strict)"("Val(Sgnl)"=FALSE ("Value (Signaling)")) -> ()  [unwired: 2 in, 2 out]
        n46 = call "Enable Output.vi"("error in (no error)"=errorcluster {"status"=FALSE, "code"=0, "source"=""}, "Enable Output  (T: Enable)"=FALSE, "VISA resource name"=w120) -> ("error out"=w118:errorcluster)  [unwired: 7 in, 1 out]
        n47 = local write "error out (Agilent)"(w118) -> ()
      }
      event "Set curet (A)", "OUTPUT": Value Change {
        n48 = event-data() -> ()  [unwired: 1 in, 3 out]
        n49 = local read "Agilent\nIntialized?"() -> (w131:bool)
        n50 = case shown="True" w131 {
          tunnel: w129 -> [_ w149]
          tunnel: [w133 w147] -> w128
          tunnel: w127 -> [w133 w146]
          tunnel: [w132 w145] -> w126
          tunnel: w125 -> [w132 w144]
          tunnel: w124 -> [_ w143]
          tunnel: w123 -> [_ w142]
          frame False {
          }
          frame True {
            w148 = u16 0 items=["Vpp", "Vrms", "dB"] ("Unit (0: Vpp)")
            w153 = u16 0 items=["DC", "Sine", "Square", "Triangle", "Ramp", "Pulse", "Noise", "Sinc", "Negative Ramp", "Exponential Rise", "Exponential Fall", "Cardiac"] ("Waveform Function (1: Sine)")
            # "To change the index to be the same as the measurement loop"
            n51 = xnode "Formula"("X1"="Set curet (A)") -> ("Result"=w150:dbl)  [unwired: 1 in, 1 out]
            n52 = Build Array (concatenate)(w144, "Set curet (A)") -> (w145:dbl[])
            n53 = Boolean To (0,1)(Boolean="OUTPUT") -> (0, 1=w136:i16)
            n54 = call "Configure Standard Waveform.vi"("Unit (0: Vpp)"=w148, "DC Offset (0.00 V)"=w150, "Frequency (1000 Hz)"=1.0, "error in (no error)"=errorcluster {"status"=FALSE, "code"=0, "source"=""}, "Amplitude (1)"=1.0, "Waveform Function (1: Sine)"=w153, "VISA resource name"=w149) -> ("error out"=w155:errorcluster, "VISA resource name out"=w156:refnum<visa-resource-name>)  [unwired: 3 in]
            n55 = Build Array(w136, "Set curet (A)") -> (w134:dbl[])
            n56 = call "Enable Output.vi"("error in (no error)"=w155, "Enable Output  (T: Enable)"="OUTPUT", "VISA resource name"=w156) -> ("error out"=w140:errorcluster)  [unwired: 7 in, 1 out]
            n57 = Get Date/Time In Seconds() -> (seconds since 1Jan1904=w138:timestamp)
            n58 = call "FileWrite.vi"("DataArray"=w134, "Time Stamp"=w138, "Error In"=w140, "FileFormat"=string[] ["%d", "%.8f"], "Index"=w142, "refnum in"=w143) -> ("Error Out"=w139:errorcluster)  [unwired: 4 in, 1 out]
            n59 = Build Array (concatenate)(w146, w138) -> (w147:timestamp[])
            n60 = local write "error out (Agilent)"(w139) -> ()
          }
        }
      }
      event "I_lim_low (A)", "I_lim_up (A)": Value Change {
        n61 = event-data() -> ()  [unwired: 1 in, 3 out]
        n62 = property on="Set curet (A)" class="DigNum (strict)"("Minimum"="I_lim_low (A)", "Maximum"="I_lim_up (A)") -> ()  [unwired: 2 in, 2 out]
      }
    }
    n63 = Equal?(x=w92, y=0) -> (x = y?=w94:bool)
    n64 = case shown="True" w94 {
      frame False {
      }
      frame True {
        n65 = local write "Graph (Set current)"(cluster{timestamp[], dbl[]} {[], []} ("Graph (Set current)")) -> ()
        "Agilent\nIntialized?" <- FALSE ("Agilent\nIntialized?")
      }
    }
    n66 = Bundle(w98, w97) -> (→"Graph (Set current)":cluster{timestamp[], dbl[]})  [unwired: 1 in]
  }
